vi "Init RT FIFOs (STM Multi-Client).vi"(8 "error in (no error)":errorcluster) -> (0 "error out":errorcluster, 3 "FIFOs out":T1 {"Data FIFO"."type" format="%0.2f"})   [LabVIEW 2019]
uses:
  RT FIFOs (STM Multi-Client).ctl
  <vilib>/real-time/rtfifo.llb/RTFIFORefnum DBLA.ctl
  <vilib>/real-time/rtfifo.llb/RTFIFORefnum BOOL.ctl
  <vilib>/real-time/NI_Real-Time Libraries.lvlib
panel:
  in  "FIFOs dummy":T1 {"Data FIFO"."type" format="%0.2f"}
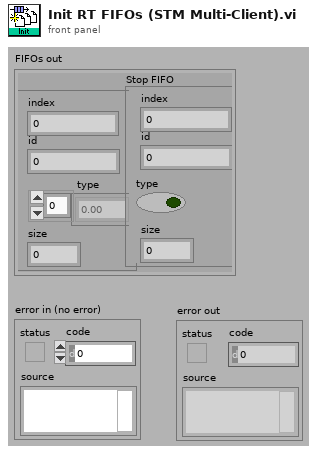
[diagram p1: front panel]
types:
  T1 = typedef "RT FIFOs (STM Multi-Client).ctl" = cluster{"Data FIFO":T2, "Stop FIFO":T3}
  T2 = typedef "NI_Real-Time Libraries.lvlib/RTFIFORefnum DBLA.ctl" = cluster{"index":u32, "id":u32, "type":dbl[], "size":u32}
  T3 = typedef "NI_Real-Time Libraries.lvlib/RTFIFORefnum BOOL.ctl" = cluster{"index":u32, "id":u32, "type":bool, "size":u32}
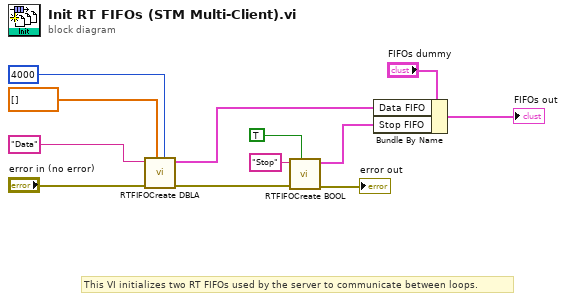
[diagram p0: block diagram]
diagram:
  # "This VI initializes two RT FIFOs used by the server to communicate between loops."
  n1 = call <vilib>:"RTFIFOCreate DBLA.vi"("elements in array (1)"=u32 4000, "type"=dbl[] [], "error in (no error)"="error in (no error)", "name (unnamed)"="Data") -> ("error out"=w9:errorcluster, "rt fifo"=w5:T2)  [unwired: 5 in, 1 out]
  n2 = call <vilib>:"RTFIFOCreate BOOL.vi"("type"=TRUE, "error in (no error)"=w9, "name (unnamed)"="Stop") -> ("error out"=→"error out":errorcluster, "rt fifo"=w6:T3)  [unwired: 6 in, 1 out]
  n3 = Bundle By Name(cluster="FIFOs dummy", "Data FIFO"=w5, "Stop FIFO"=w6) -> (→"FIFOs out":T1)
